vi "Get Variant Message.vi"(8 "error in (no error)":errorcluster, 11 "Car Out of Position in":refnum<class "Car Out of Position.lvclass">) -> (0 "error out":errorcluster, 1 "Value":variant, 2 "Name":string, 3 "Car Out of Position out":refnum<class "Car Out of Position.lvclass">)   [LabVIEW 2016, in "CLD Exam - Car Wash.lvlib" / "Car Out of Position.lvclass"]
doc: "--\nCopyright © 2017 Composed SystemsI All rights reserved.\n\nAuthor: Jon McBee <jon.mcbee@composed.io>\n\nThis library is provided \"AS IS\" ,WITHOUT WARRANTIES OR\nCONDITIONS OF ANY KIND, either express or implied.\n\nComposed Systems -- composed.io\n\nStream 0.0.1.1\nJon McBee - Composed Systems\nCopyright (c) 2017, Composed Systems"
uses:
  Car Out of Position.lvclass
  Mediator/Classes/Message Data Interface/Data Message Interface.lvclass
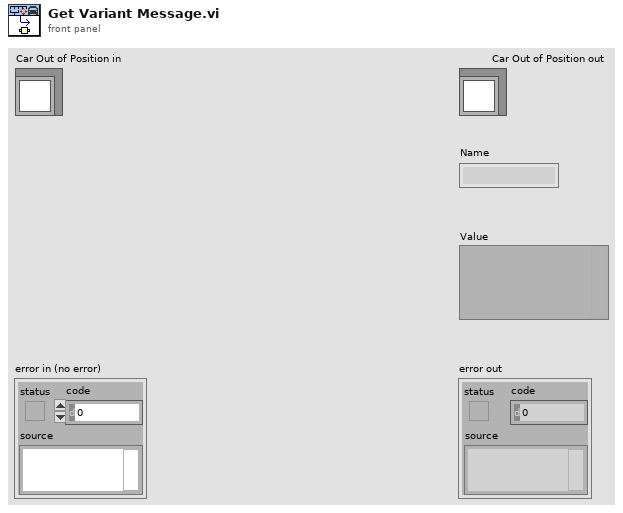
[diagram p1: front panel]
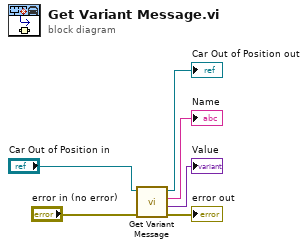
[diagram p0: block diagram]
diagram:
  n1 = call-parent "Get Variant Message.vi"("error in (no error)"="error in (no error)", "Data Message Interface in"="Car Out of Position in") -> ("error out"=→"error out":errorcluster, "Value"=→"Value":variant, "Name"=→"Name":string, "Data Message Interface out"=→"Car Out of Position out":refnum<class "Car Out of Position.lvclass">)  [unwired: 6 in]
